vi "PUMP RAMP (SubVI).vi"(0 "Dynamic Data":dynamicdata(waveform), 1 "Numeric":i16, 3 "Seq in":dbl[][](array[numeric])=[[20.0, 60.0, 40.0], [60.0, 40.0, 20.0], [100.0, 100.0, 100.0]], 5 "?":bool, 6 "bypass":bool, 8 "bypass RPM":dbl) -> (7 "Rate (g/s)":dbl, 10 "Weight (S1)":dbl, 11 "Step 2":i32, 12 "target reached":i32, 13 "x/y":dbl, 14 "Time (s)":dbl, 15 "bal_previous":i32, 17 "Target (g)":dbl, 18 "Waveform Chart 2":dynamicdata(graph), 19 "DAQ assistant (4-20 mA)":dbl)   [LabVIEW 2015]
uses:
  x64/Debug/BERTTA.dll
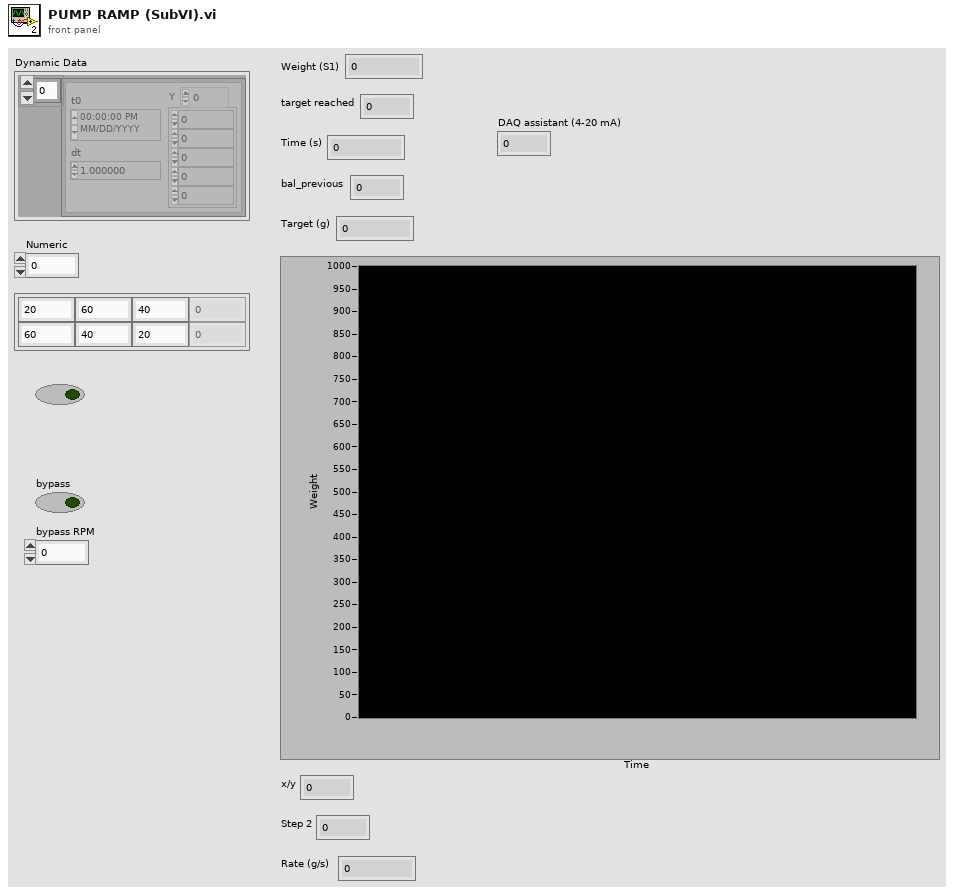
[diagram p1: front panel]
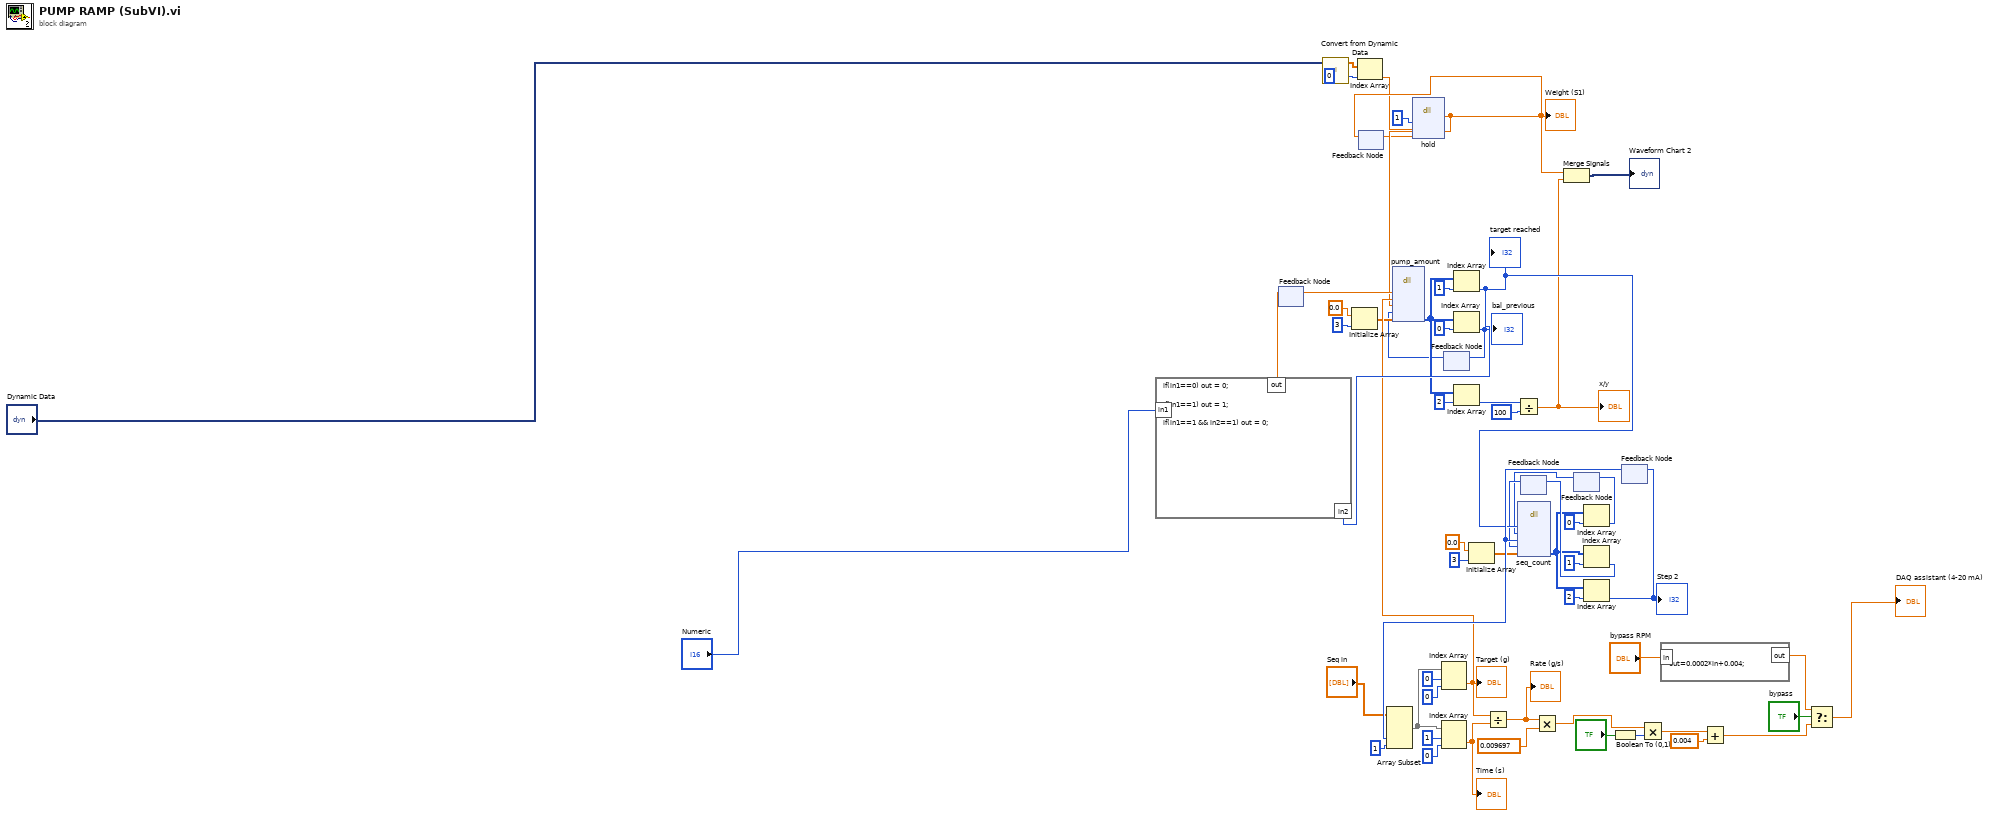
[diagram p0: block diagram]
diagram:
  n1 = feedback #1() -> (w55:dbl)  [unwired: 1 in]
  n2 = call "Convert from Dynamic Data"("Dynamic Data Type"="Dynamic Data") -> ("Array"=w22:dbl[])  [unwired: 3 in]
  n3 = Initialize Array(0.0 ("element"), 3 ("dimension size")) -> (w32:dbl[])
  n4 = Index Array(array=w22, index=0) -> (element=w23:dbl)
  n5 = feedback #2() -> (w24:dbl)  [unwired: 1 in]
  n6 = dll-call lib="C:/Users/shresplab/OneDrive - Kemira Oyj/Documents/Visual Studio 2017/Projects/Bertta/BERTTA/x64/Debug/BERTTA.dll" fn="hold"("enable"=1, "in1"=w23, "in2"=w24) -> ("return type"=w35:dbl)  [unwired: 6 in, 2 out]
  "Weight (S1)" <- w35
  n7 = feedback-in #2(w35) -> ()
  n8 = feedback #3() -> (w29:i32)  [unwired: 1 in]
  n9 = Initialize Array(0.0 ("element"), 3 ("dimension size")) -> (w41:dbl[])
  n10 = feedback #4() -> (w49:i32)  [unwired: 1 in]
  n11 = feedback #5() -> (w48:i32)  [unwired: 1 in]
  n12 = Boolean To (0,1)(Boolean="?") -> (0, 1=w9:i16)
  n13 = feedback #6() -> (w57:i32)  [unwired: 1 in]
  n14 = Array Subset(array="Seq in", index (col)=w57, length (col)=1 ("length")) -> (w13:dbl[][])  [unwired: 2 in]
  n15 = Index Array(array=w13, index (row)=0, index (col)=0 ("disabled index (col)")) -> (element=w37:dbl)
  "Target (g)" <- w37
  n16 = dll-call lib="C:/Users/shresplab/OneDrive - Kemira Oyj/Documents/Visual Studio 2017/Projects/Bertta/BERTTA/x64/Debug/BERTTA.dll" fn="pump_amount"("enable"=w55, "target"=w37, "bal"=w35, "bal_previous"=w29, "params"=w32) -> ("params"=w34:i32[])  [unwired: 8 in, 2 out]
  n17 = Index Array(array=w13, index (row)=1, index (col)=0 ("disabled index (col)")) -> (element=w17:dbl)
  "Time (s)" <- w17
  n18 = Index Array(array=w34, index=1) -> (element=w53:i32)
  "target reached" <- w53
  n19 = formula code="if(in1==0) out = 0;\n\nif(in1==1) out = 1;\n\nif(in1==1 && in2==1) out = 0;"("in1"="Numeric", "in2"=w53) -> ("out"=w54:dbl)
  n20 = feedback-in #1(w54) -> ()
  n21 = Index Array(array=w34, index=0) -> (element=w28:i32)
  "bal_previous" <- w28
  n22 = feedback-in #3(w28) -> ()
  n23 = Index Array(array=w34, index=2) -> (element=w38:i32)
  n24 = Divide(x=w37, y=w17) -> (x/y=w18:dbl)
  "Rate (g/s)" <- w18
  n25 = Divide(x=w38, y=100) -> (x/y=w39:dbl)
  "x/y" <- w39
  n26 = dll-call lib="C:/Users/shresplab/OneDrive - Kemira Oyj/Documents/Visual Studio 2017/Projects/Bertta/BERTTA/x64/Debug/BERTTA.dll" fn="seq_count"("in1"=w53, "in2"=w48, "in3"=w57, "in4"=w49, "params"=w41) -> ("params"=w47:i32[])  [unwired: 8 in, 2 out]
  n27 = Multiply(x=w18, y=0.009697) -> (x*y=w7:dbl)
  n28 = Merge Signals(w35, w39) -> (→"Waveform Chart 2":dynamicdata)
  n29 = Index Array(array=w47, index=0) -> (element=w50:i32)
  n30 = feedback-in #5(w50) -> ()
  n31 = Index Array(array=w47, index=1) -> (element=w51:i32)
  n32 = feedback-in #4(w51) -> ()
  n33 = Index Array(array=w47, index=2) -> (element=w56:i32)
  "Step 2" <- w56
  n34 = feedback-in #6(w56) -> ()
  n35 = Multiply(x=w7, y=w9) -> (x*y=w6:dbl)
  n36 = formula code="out=0.0002*in+0.004;"("in"="bypass RPM") -> ("out"=w2:dbl)
  n37 = Add(x=w6, y=0.004) -> (x+y=w3:dbl)
  n38 = Select(t=w2, s="bypass", f=w3) -> (s? t:f=→"DAQ assistant (4-20 mA)":dbl)
